vi "Read Stage Position.vi"(4 "error in":errorcluster, 5 "VISA resource name in":refnum<visa-resource-name>) -> (0 "Current Position":cluster{dbl, dbl, dbl}, 1 "error out":errorcluster, 2 "VISA resource name out":refnum<visa-resource-name>)   [LabVIEW 2016]
uses:
  <vilib>/Instr/_visa.llb/VISA Configure Serial Port (Instr).vi
panel:
  out "Serial Settings:Number of Bytes at Serial Port":u32
  out "read buffer":string
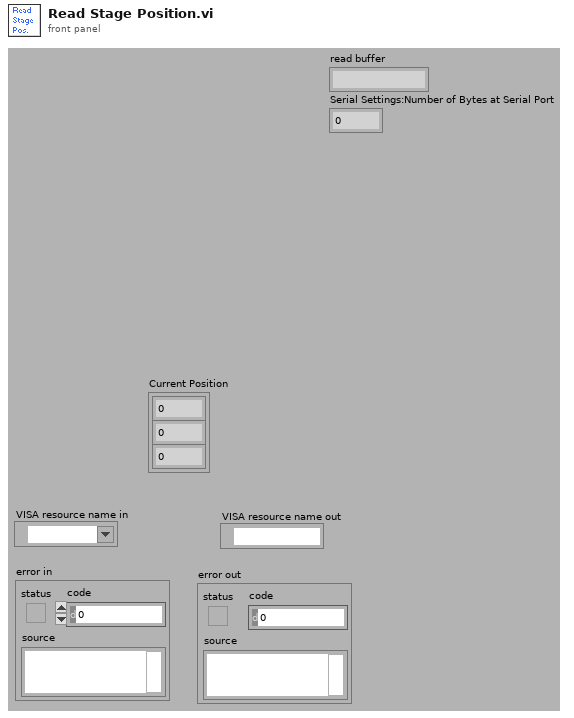
[diagram p1: front panel]
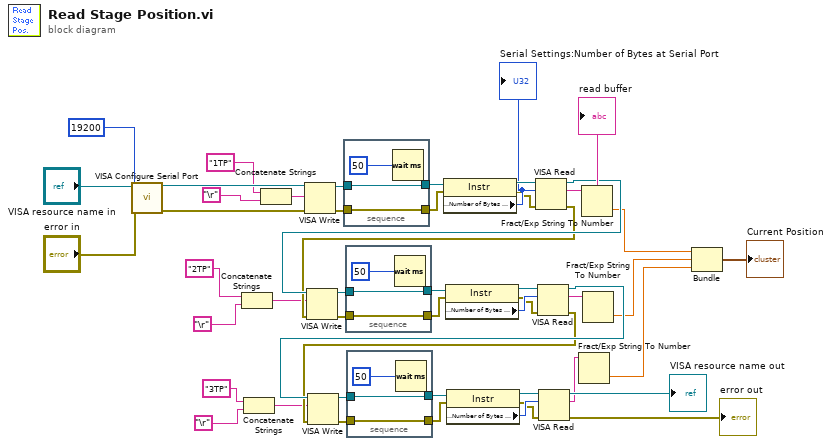
[diagram p0: block diagram]
diagram:
  n1 = call-poly "VISA Configure Serial Port"("VISA resource name"="VISA resource name in", "baud rate (9600)"=u32 19200, "error in (no error)"="error in") -> ("VISA resource name out"=w45:refnum<visa-resource-name>, "error out"=w44:errorcluster)  [unwired: 3 in, 8 out]
  n2 = Concatenate Strings("2TP" ("write buffer"), "\r") -> (w11:string)
  n3 = Concatenate Strings("3TP" ("write buffer"), "\r") -> (w9:string)
  n4 = Concatenate Strings("1TP" ("write buffer"), "\r") -> (w12:string)
  n5 = VISA Write(VISA resource name=w45, write buffer=w12, error in (no error)=w44) -> (VISA resource name out=w41:refnum<visa-resource-name>, error out=w40:errorcluster)  [unwired: 1 out]
  n6 = stacked-sequence {
    tunnel: [w51] -> w39
    tunnel: w41 -> [w51]
    tunnel: w40 -> [w50]
    tunnel: [w50] -> w34
    frame #0 {
      n7 = Wait (ms)(milliseconds to wait=50) -> ()  [unwired: 1 out]
    }
  }
  n8 = property class="Instr"(reference=w39, error in=w34) -> (reference out=w38:refnum<visa-resource-name>, error out=w36:errorcluster, "Serial Settings:Number of Bytes at Serial Port"=w37:u32)
  "Serial Settings:Number of Bytes at Serial Port" <- w37
  n9 = VISA Read(VISA resource name=w38, byte count=w37, error in (no error)=w36) -> (VISA resource name out=w17:refnum<visa-resource-name>, read buffer=w35:string, error out=w15:errorcluster)  [unwired: 1 out]
  "read buffer" <- w35
  n10 = VISA Write(VISA resource name=w17, write buffer=w11, error in (no error)=w15) -> (VISA resource name out=w33:refnum<visa-resource-name>, error out=w32:errorcluster)  [unwired: 1 out]
  n11 = stacked-sequence {
    tunnel: [w54] -> w31
    tunnel: w33 -> [w54]
    tunnel: w32 -> [w53]
    tunnel: [w53] -> w26
    frame #0 {
      n12 = Wait (ms)(milliseconds to wait=50) -> ()  [unwired: 1 out]
    }
  }
  n13 = property class="Instr"(reference=w31, error in=w26) -> (reference out=w30:refnum<visa-resource-name>, error out=w28:errorcluster, "Serial Settings:Number of Bytes at Serial Port"=w29:u32)
  n14 = VISA Read(VISA resource name=w30, byte count=w29, error in (no error)=w28) -> (VISA resource name out=w16:refnum<visa-resource-name>, read buffer=w27:string, error out=w14:errorcluster)  [unwired: 1 out]
  n15 = VISA Write(VISA resource name=w16, write buffer=w9, error in (no error)=w14) -> (VISA resource name out=w25:refnum<visa-resource-name>, error out=w24:errorcluster)  [unwired: 1 out]
  n16 = stacked-sequence {
    tunnel: [w57] -> w23
    tunnel: w25 -> [w57]
    tunnel: w24 -> [w56]
    tunnel: [w56] -> w18
    frame #0 {
      n17 = Wait (ms)(milliseconds to wait=50) -> ()  [unwired: 1 out]
    }
  }
  n18 = property class="Instr"(reference=w23, error in=w18) -> (reference out=w22:refnum<visa-resource-name>, error out=w20:errorcluster, "Serial Settings:Number of Bytes at Serial Port"=w21:u32)
  n19 = VISA Read(VISA resource name=w22, byte count=w21, error in (no error)=w20) -> (VISA resource name out=→"VISA resource name out":refnum<visa-resource-name>, read buffer=w19:string, error out=→"error out":errorcluster)  [unwired: 1 out]
  n20 = Fract/Exp String To Number(string=w19) -> (number=w5:dbl)  [unwired: 4 out]
  n21 = Fract/Exp String To Number(string=w35) -> (number=w7:dbl)  [unwired: 4 out]
  n22 = Fract/Exp String To Number(string=w27) -> (number=w6:dbl)  [unwired: 4 out]
  n23 = Bundle(w7, w6, w5) -> (→"Current Position":cluster{dbl, dbl, dbl})  [unwired: 1 out]
